vi "FixWorldToHoriz.vi"(1 "Stage In":refnum<vi>) -> (0 "Scene.Object Out":refnum<vi>)   [LabVIEW 2010]
uses:
  <vilib>/picture/3D Picture Control/NI_3D Picture Control.lvlib
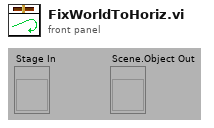
[diagram p1: front panel]
types:
  T1 = cluster{"Final Zoom":sgl, "Final Zoom":sgl, "Resolution":i32}
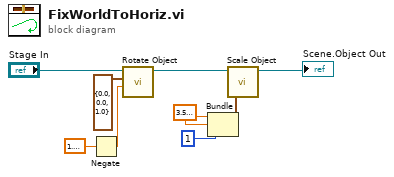
[diagram p0: block diagram]
diagram:
  w5 = sgl 3.6 ("Final Zoom")
  n1 = Negate(x=1.5707963267948966) -> (-x=w6:dbl)
  n2 = call <vilib>:"Rotate Object.vi"("Angle"=w6, "Axis"=cluster{"X":sgl, "Y":sgl, "Z":sgl} {"X"=0.0, "Y"=0.0, "Z"=1.0}, "Scene.Object In"="Stage In") -> ("Scene.Object Out"=w2:refnum<vi>)  [unwired: 7 in, 1 out]
  n3 = Bundle("Final Zoom"=w5, "Final Zoom"=w5, "Resolution"=1) -> (w3:T1)  [unwired: 1 in]
  n4 = call <vilib>:"Scale Object.vi"("Scale"=w3, "Scene.Object In"=w2) -> ("Scene.Object Out"=→"Scene.Object Out":refnum<vi>)  [unwired: 8 in, 1 out]
